vi "XNET String To IO Name (Signal).vi"(3 "string":string) -> (0 "XNET Signal":refnum<k21>)   [LabVIEW 2018]
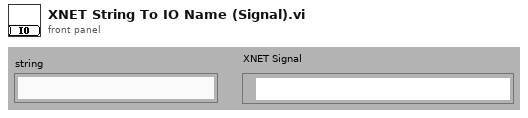
[diagram p1: front panel]
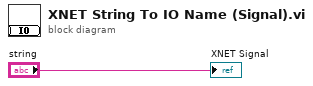
[diagram p0: block diagram]
diagram:
  "XNET Signal" <- "string"
